vi "test.vi"() -> ()   [LabVIEW 2016]
panel:
  out "AI0":dbl
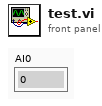
[diagram p1: front panel]
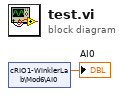
[diagram p0: block diagram]
diagram:
  n1 = shared-variable "cRIO1-WinklerLab\\Mod6\\AI0"() -> (→"AI0":dbl)  [unwired: 1 in, 1 out]
